vi "Vision Processing.vi"() -> ()   [LabVIEW 2011]
doc: "This VI runs in parallel to other tasks. It gets images from the camera, processes them for color or shape and use that information to affect robot behavior."
uses:
  Robot Global Data.vi
  <vilib>/vision/NI_Vision_Development_Module.lvlib
panel:
  in  "Lower Speed Limit":dbl=0.05
  in  "Score Limits":T1={"Rect Coverage"=76.0, "Aspect Ratio"=40.0, "X Edge Strength"=40.0, "Y Edge Strength"=60.0}
  out "Processed Image":T2(plugin-control)
  out "Original Image":T2(plugin-control)
  in  "Annotate":bool=TRUE
  in  "Particle Count Limit":i32=10
  in  "Area Size Limit":i32=444
  in  "Range":cluster{"Lower value":sgl, "Upper value":sgl}={"Lower value"=120.0, "Upper value"=255.0}
  out "X Position Array":dbl[](array[numeric])
  out "Y Position Array":dbl[](array[numeric])
  out "Number of Rectangles Visible":dbl
  in  "Upper Speed Limit":dbl=0.3
  out "Turret Rotation":dbl
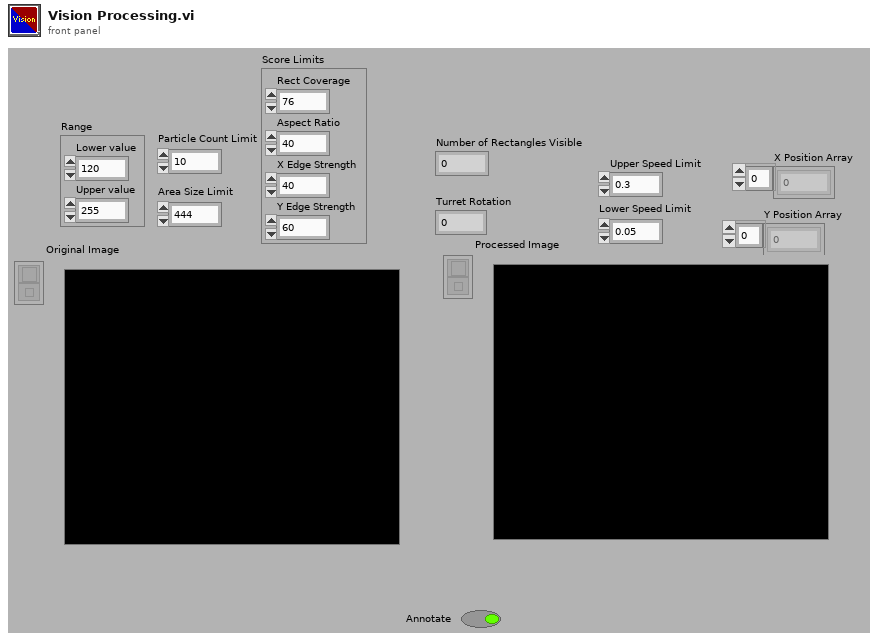
[diagram p1: front panel]
types:
  T1 = cluster{"Rect Coverage":dbl, "Aspect Ratio":dbl, "X Edge Strength":dbl, "Y Edge Strength":dbl}
  T2 = typedef "IMAQ Image.ctl" = refnum<image>
  T3 = typedef "Image Type" = u32
  T4 = typedef "WPI_CameraImageSize.ctl" = enum16{"640x480", "320x240", "160x120"}
  T5 = cluster{"fps":i32, "compression":i32, "Image Size":T4}
  T6 = cluster{"Position":cluster{"X":dbl, "Y":dbl}, "Distance (ft)":dbl}[]
  T7 = cluster{cluster{"Left":dbl, "Top":dbl, "Right":dbl, "Bottom":dbl}, dbl[]}[]
  T8 = cluster{"Left":dbl, "Top":dbl, "Right":dbl, "Bottom":dbl}
  T9 = cluster{"Target Center (-1 to 1)":cluster{"X":dbl, "Y":dbl}, "Distance (ft)":dbl}
  T10 = cluster{"Target Center (-1 to 1)":cluster{"X":dbl, "Y":dbl}, "Distance (ft)":dbl}[]
  T11 = cluster{"Axis 1":dbl, "Axis 2":dbl, "Axis 3":dbl, "Axis 4":dbl, "Axis 5":dbl, "Axis 6":dbl, "Button 1":bool, "Button 2":bool, "Button 3":bool, "Button 4":bool, "Button 5":bool, "Button 6":bool, "Button 7":bool, "Button 8":bool, "Button 9":bool, "Button 10":bool, "Button 11":bool, "Button 12":bool}
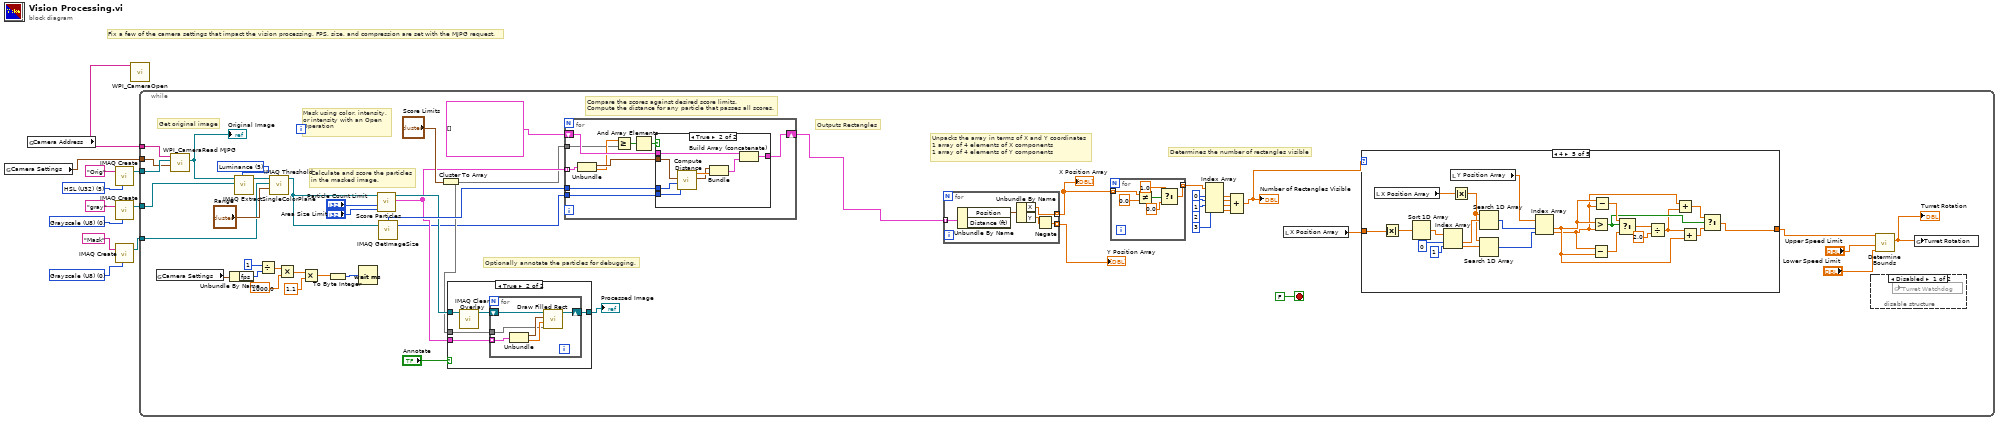
[diagram p0: block diagram]
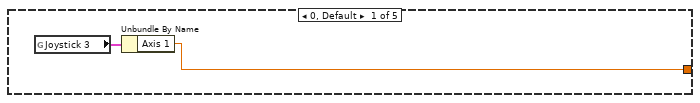
[diagram p3: hidden frame]
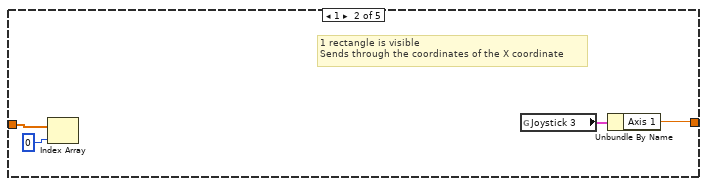
[diagram p4: hidden frame]
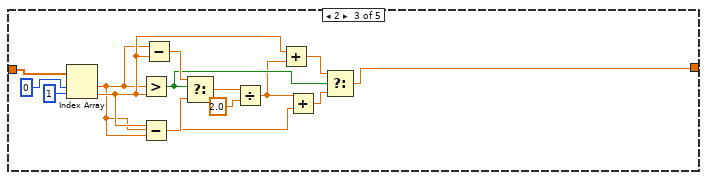
[diagram p5: hidden frame]
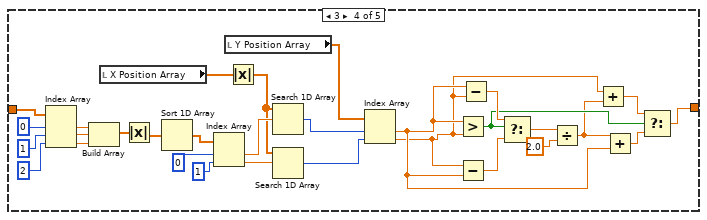
[diagram p6: hidden frame]
diagram:
  w4 = T3 0 items=["Grayscale (U8)", "Grayscale (I16)", "Grayscale (SGL)", "Complex (CSG)", "RGB (U32)", "HSL (U32)", "RGB (U64)", "Grayscale (U16)"] ("Image Type")
  w8 = T3 5 items=["Grayscale (U8)", "Grayscale (I16)", "Grayscale (SGL)", "Complex (CSG)", "RGB (U32)", "HSL (U32)", "RGB (U64)", "Grayscale (U16)"] ("Image Type")
  w11 = T3 0 items=["Grayscale (U8)", "Grayscale (I16)", "Grayscale (SGL)", "Complex (CSG)", "RGB (U32)", "HSL (U32)", "RGB (U64)", "Grayscale (U16)"] ("Image Type")
  # "Fix a few of the camera settings that impact the vision processing. FPS, size, and compression are set with the MJPG request."
  n1 = global read "Robot Global Data.vi" "Camera Settings"() -> (w1:T5)
  n2 = global read "Robot Global Data.vi" "Camera Address"() -> (w2:string)
  n3 = call "IMAQ Create"("Image Name"="Orig", "Image Type"=w8) -> ("New Image"=w7:T2)  [unwired: 2 in, 2 out]
  n4 = call "IMAQ Create"("Image Name"="gray", "Image Type"=w11) -> ("New Image"=w6:T2)  [unwired: 2 in, 2 out]
  n5 = call "IMAQ Create"("Image Name"="Mask", "Image Type"=w4) -> ("New Image"=w3:T2)  [unwired: 2 in, 2 out]
  n6 = call <vilib>:"WPI_CameraOpen.vi"("Camera Address"=w2) -> ()  [unwired: 9 in, 2 out]
  n7 = while {
    tunnel: w7 -> [w59]
    tunnel: w6 -> [w41]
    tunnel: w3 -> [w43]
    tunnel: w2 -> [w58]
    tunnel: w1 -> [w47]
    stop <- FALSE stop-if-true
    w46 = 5 items=["Red", "Green", "Blue", "Hue", "Saturation", "Luminance", "Value", "Intensity"] ("Color Plane")
    # "Outputs Rectangles"
    # "Determines the number of rectangles visible"
    # "Unpacks the array in terms of X and Y coordinates\n1 array of 4 elements of X components\n1 array of 4 elements of Y components"
    # "Optionally annotate the particles for debugging."
    # "Compare the scores against desired score limits.\nCompute the distance for any particle that passes all scores."
    # "Calculate and score the particles\nin the masked image."
    # "Mask using color, intensity,\nor intensity with an Open\nOperation"
    # "Get original image"
    n8 = global read "Robot Global Data.vi" "Camera Settings"() -> (w24:T5)
    n9 = call <vilib>:"WPI_CameraRead MJPG.vi"("Camera Settings"=w47, "Image"=w59, "address"=w58) -> ("Image Out"=w42:T2)  [unwired: 7 in, 1 out]
    "Original Image" <- w42
    n10 = Unbundle By Name(w24) -> ("fps"=w23:i32)
    n11 = call "IMAQ ExtractSingleColorPlane"("Color Plane"=w46, "Image Dst"=w41, "Image Src"=w42) -> ("Image Dst Out"=w44:T2)  [unwired: 1 in, 7 out]
    n12 = Divide(x=1, y=w23) -> (x/y=w21:dbl)
    n13 = call "IMAQ Threshold"("Range"="Range", "Image Dst"=w43, "Image Src"=w44) -> ("Image Dst Out"=w40:T2)  [unwired: 3 in, 5 out]
    n14 = Multiply(x=w21, y=1000.0) -> (x*y=w19:dbl)
    n15 = Multiply(x=w19, y=1.1) -> (x*y=w17:dbl)
    n16 = To Byte Integer(number=w17) -> (8bit integer=w16:i8)
    n17 = Wait (ms)(milliseconds to wait=w16) -> ()  [unwired: 1 out]
    n18 = call "Score Particles.vi"("Area Size Limit"="Area Size Limit", "Particle Count Limit"="Particle Count Limit", "Image Refnum in"=w40) -> ("Scored Particle Info"=w54:T7, "Image Refnum out"=w57:T2)  [unwired: 7 in]
    n19 = call "IMAQ GetImageSize"("Image"=w40) -> ("Y Resolution"=w48:i32, "X Resolution"=w60:i32)  [unwired: 3 in, 1 out]
    n20 = Cluster To Array(cluster="Score Limits") -> (array=w52:dbl[])
    n21 = case shown="True" "Annotate" {
      tunnel: w57 -> [w145 w150]
      tunnel: [w145 w149] -> w55
      tunnel: w54 -> [_ w147]
      tunnel: w52 -> [_ w146]
      frame False {
      }
      frame True {
        n22 = call "IMAQ Clear Overlay"("Image"=w150) -> ("Image Out"=w148:T2)  [unwired: 2 in, 8 out]
        n23 = for {
          shift-right: [w155] -> w149
          shift-left: w148 -> [w156]
          tunnel: w147 -> [w152] mode=indexing
          tunnel: w146 -> [w151]
          n24 = Unbundle(w152) -> (w153:T8, w154:dbl[])
          n25 = call "Draw Filled Rect.vi"("Limits"=w151, "Scores"=w154, "Bounding Box"=w153, "image in"=w156) -> ("image out"=w155:T2)  [unwired: 7 in]
        }
      }
    }
    "Processed Image" <- w55
    n26 = for {
      shift-right: [w165] -> w26
      shift-left: T6 [] -> [w166]
      tunnel: w60 -> [w164]
      tunnel: w54 -> [w162] mode=indexing
      tunnel: w52 -> [w158]
      tunnel: w48 -> [w157]
      n27 = Unbundle(w162) -> (w163:T8, w159:dbl[])
      n28 = Greater Or Equal?(x=w159, y=w158) -> (x >= y?=w161:bool[])
      n29 = And Array Elements(Boolean array=w161) -> (logical AND=w160:bool)
      n30 = case shown="True" w160 {
        tunnel: w166 -> [w167 w175]
        tunnel: [w167 w174] -> w165
        tunnel: w163 -> [_ w170]
        tunnel: w164 -> [_ w172]
        tunnel: w157 -> [_ w168]
        frame False {
        }
        frame True {
          n31 = call "Compute Distance.vi"("Y Image Resolution"=w168, "X Image Resolution"=w172, "Bounding Box"=w170) -> ("Target Center (-1 to 1)"=w169:cluster{"X":dbl, "Y":dbl}, "Distance (ft)"=w171:dbl)  [unwired: 7 in]
          n32 = Bundle("Target Center (-1 to 1)"=w169, "Distance (ft)"=w171) -> (w173:T9)  [unwired: 1 in]
          n33 = Build Array (concatenate)(w175, w173) -> (w174:T10)
        }
      }
    }
    n34 = for {
      tunnel: [w141] -> w25 mode=indexing
      tunnel: [w143] -> w38 mode=indexing
      tunnel: w26 -> [w142] mode=indexing
      n35 = Unbundle By Name(w142) -> ("Position"=w144:cluster{"X":dbl, "Y":dbl})  [unwired: 1 out]
      n36 = Unbundle By Name(w144) -> ("X"=w143:dbl, "Y"=w140:dbl)
      n37 = Negate(x=w140) -> (-x=w141:dbl)
    }
    "X Position Array" <- w38
    "Y Position Array" <- w25
    n38 = for {
      tunnel: w38 -> [w65] mode=indexing
      tunnel: [w61] -> w37 mode=indexing
      n39 = Not Equal?(x=w65, y=0.0) -> (x != y?=w64:bool)
      n40 = Select(t=1.0, s=w64, f=0.0) -> (s? t:f=w61:dbl)
    }
    n41 = Index Array(array=w37, index #1=0 ("index"), index #2=1 ("index"), index #3=2 ("index"), index #4=3 ("index")) -> (element #1=w35:dbl, element #2=w36:dbl, element #3=w34:dbl, element #4=w33:dbl)
    n42 = Compound Arithmetic op=ADD(w35, w36, w34, w33) -> (w27:dbl)
    "Number of Rectangles Visible" <- w27
    n43 = local read "X Position Array"() -> (w39:dbl[])
    n44 = case shown="4" w27 {
      tunnel: w39 -> [_ w72 w86 w116 w119]
      tunnel: [w67 w69 w73 w88 w118] -> w12
      frame 0, Default {
        n45 = global read "Robot Global Data.vi" "Joystick 3"() -> (w68:T11)
        n46 = Unbundle By Name(w68) -> ("Axis 1"=w67:dbl)
      }
      frame 1 {
        # "1 rectangle is visible\nSends through the coordinates of the X coordinate"
        n47 = Index Array(array=w72, index=0) -> ()  [unwired: 1 out]
        n48 = global read "Robot Global Data.vi" "Joystick 3"() -> (w70:T11)
        n49 = Unbundle By Name(w70) -> ("Axis 1"=w69:dbl)
      }
      frame 2 {
        n50 = Index Array(array=w86, index #1=0 ("index"), index #2=1 ("index")) -> (element #1=w74:dbl, element #2=w75:dbl)
        n51 = Greater?(x=w74, y=w75) -> (0:w79:bool)
        n52 = Subtract(x=w75, y=w74) -> (x-y=w82:dbl)
        n53 = Subtract(x=w74, y=w75) -> (x-y=w83:dbl)
        n54 = Select(t=w83, s=w79, f=w82) -> (s? t:f=w81:dbl)
        n55 = Divide(x=w81, y=2.0) -> (x/y=w76:dbl)
        n56 = Add(x=w75, y=w76) -> (x+y=w78:dbl)
        n57 = Add(x=w76, y=w74) -> (x+y=w77:dbl)
        n58 = Select(t=w78, s=w79, f=w77) -> (s? t:f=w73:dbl)
      }
      frame 3 {
        n59 = Index Array(array=w116, index #1=0 ("index"), index #2=1 ("index"), index #3=2 ("index")) -> (element #1=w112:dbl, element #2=w111:dbl, element #3=w110:dbl)
        n60 = Build Array(w112, w111, w110) -> (w109:dbl[])
        n61 = local read "X Position Array"() -> (w102:dbl[])
        n62 = Absolute Value(x=w109) -> (abs(x)=w108:dbl[])
        n63 = Sort 1D Array(array=w108) -> (sorted array=w107:dbl[])
        n64 = Index Array(array=w107, index #1=0 ("index"), index #2=1 ("index")) -> (element #1=w104:dbl, element #2=w103:dbl)
        n65 = local read "Y Position Array"() -> (w100:dbl[])
        n66 = Absolute Value(x=w102) -> (abs(x)=w87:dbl[])
        n67 = Search 1D Array(1D array=w87, element=w104) -> (index of element=w101:i32)  [unwired: 1 in]
        n68 = Search 1D Array(1D array=w87, element=w103) -> (index of element=w99:i32)  [unwired: 1 in]
        n69 = Index Array(array=w100, index #1=w101, index #2=w99) -> (element #1=w90:dbl, element #2=w89:dbl)
        n70 = Greater?(x=w90, y=w89) -> (0:w94:bool)
        n71 = Subtract(x=w89, y=w90) -> (x-y=w97:dbl)
        n72 = Subtract(x=w90, y=w89) -> (x-y=w98:dbl)
        n73 = Select(t=w98, s=w94, f=w97) -> (s? t:f=w96:dbl)
        n74 = Divide(x=w96, y=2.0) -> (x/y=w91:dbl)
        n75 = Add(x=w89, y=w91) -> (x+y=w93:dbl)
        n76 = Add(x=w91, y=w90) -> (x+y=w92:dbl)
        n77 = Select(t=w93, s=w94, f=w92) -> (s? t:f=w88:dbl)
      }
      frame 4 {
        n78 = local read "X Position Array"() -> (w133:dbl[])
        n79 = Absolute Value(x=w119) -> (abs(x)=w139:dbl[])
        n80 = Sort 1D Array(array=w139) -> (sorted array=w138:dbl[])
        n81 = Index Array(array=w138, index #1=0 ("index"), index #2=1 ("index")) -> (element #1=w135:dbl, element #2=w134:dbl)
        n82 = local read "Y Position Array"() -> (w131:dbl[])
        n83 = Absolute Value(x=w133) -> (abs(x)=w117:dbl[])
        n84 = Search 1D Array(1D array=w117, element=w135) -> (index of element=w132:i32)  [unwired: 1 in]
        n85 = Search 1D Array(1D array=w117, element=w134) -> (index of element=w130:i32)  [unwired: 1 in]
        n86 = Index Array(array=w131, index #1=w132, index #2=w130) -> (element #1=w121:dbl, element #2=w120:dbl)
        n87 = Greater?(x=w121, y=w120) -> (0:w125:bool)
        n88 = Subtract(x=w120, y=w121) -> (x-y=w128:dbl)
        n89 = Subtract(x=w121, y=w120) -> (x-y=w129:dbl)
        n90 = Select(t=w129, s=w125, f=w128) -> (s? t:f=w127:dbl)
        n91 = Divide(x=w127, y=2.0) -> (x/y=w122:dbl)
        n92 = Add(x=w120, y=w122) -> (x+y=w124:dbl)
        n93 = Add(x=w122, y=w121) -> (x+y=w123:dbl)
        n94 = Select(t=w124, s=w125, f=w123) -> (s? t:f=w118:dbl)
      }
    }
    n95 = disable-structure shown="Disabled" {
      frame Disabled {
        n96 = global read "Robot Global Data.vi" "Turret Watchdog"() -> ()  [unwired: 1 in]
      }
      frame Enabled {
      }
    }
    n97 = call "Determine Bounds.vi"("Lower Limit"="Lower Speed Limit", "Upper Limit"="Upper Speed Limit", "Input"=w12) -> ("Output"=w13:dbl)  [unwired: 8 in]
    "Turret Rotation" <- w13
    n98 = global write "Robot Global Data.vi" "Turret Rotation"(w13) -> ()
  }
